vi "Testing-mydaq.vi"() -> ()   [LabVIEW 2020]
uses:
  <vilib>/DAQmx/read.llb/DAQmx Read (Analog 1D DBL 1Chan NSamp).vi
  <vilib>/DAQmx/create/channels.llb/DAQmx Create Channel (AI-Voltage-Basic).vi
  <vilib>/DAQmx/configure/timing.llb/DAQmx Timing (Sample Clock).vi
  <vilib>/DAQmx/miscellaneous.llb/DAQmx Fill In Error Info.vi
panel:
  out "Waveform Chart":dbl[](graph)
  in  "stop":bool
  out "error out":errorcluster
  out "data":dbl[](array[numeric]) format="%0.2f"
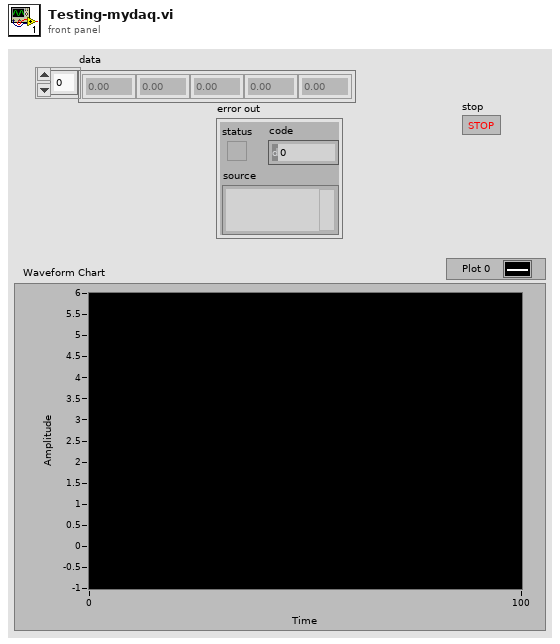
[diagram p1: front panel]
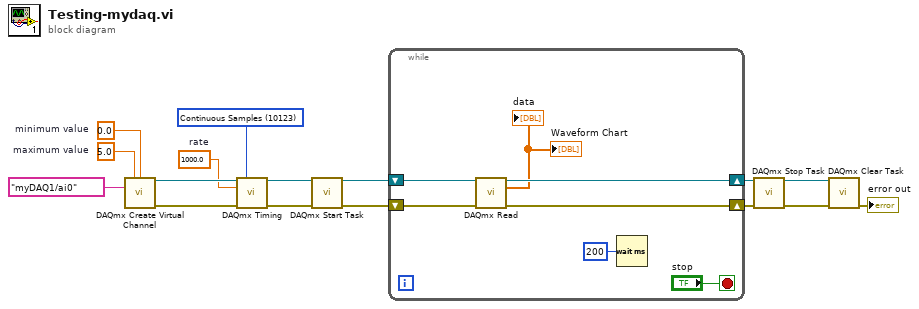
[diagram p0: block diagram]
diagram:
  w8 = 10123 items=["Finite Samples"=10178, "Continuous Samples"=10123, "Hardware Timed Single Point"=12522] ("sample mode")
  w11 = 1000.0  # rate
  w14 = 0.0  # minimum value
  w15 = 5.0  # maximum value
  n1 = call-poly <vilib>:"DAQmx Create Virtual Channel.vi"("maximum value"=w15, "minimum value"=w14, "physical channels"=tag "myDAQ1/ai0") -> ("task out"=w13:refnum<k21>, "error out"=w12:errorcluster)  [unwired: 11 in]
  n2 = call-poly <vilib>:"DAQmx Timing.vi"("task/channels in"=w13, "sample mode"=w8, "rate"=w11, "error in"=w12) -> ("task out"=w10:refnum<k21>, "error out"=w9:errorcluster)  [unwired: 10 in]
  n3 = call <vilib>:"DAQmx Start Task.vi"("task/channels in"=w10, "error in"=w9) -> ("task out"=w7:refnum<k21>, "error out"=w6:errorcluster)  [unwired: 12 in]
  n4 = while {
    shift-right: [w21] -> w5
    shift-left: w7 -> [w23]
    shift-right: [w20] -> w2
    shift-left: w6 -> [w22]
    stop <- "stop" stop-if-true
    n5 = call-poly <vilib>:"DAQmx Read.vi"("task/channels in"=w23, "error in"=w22) -> ("task out"=w21:refnum<k21>, "data"=→"data" →"Waveform Chart":dbl[], "error out"=w20:errorcluster)  [unwired: 11 in]
    n6 = Wait (ms)(milliseconds to wait=u32 200) -> ()  [unwired: 1 out]
  }
  n7 = call <vilib>:"DAQmx Stop Task.vi"("task/channels in"=w5, "error in"=w2) -> ("task out"=w4:refnum<k21>, "error out"=w3:errorcluster)  [unwired: 12 in]
  n8 = call <vilib>:"DAQmx Clear Task.vi"("task in"=w4, "error in"=w3) -> ("error out"=→"error out":errorcluster)  [unwired: 13 in]
